vi "MQTT_PingReq.vi"(8 "error in (no error)":errorcluster, 11 "SSL_Connection":T1) -> (0 "error out":errorcluster, 2 "PingReq Message":u8[](array[numeric]) format="%x", 3 "SSL_Connection":T1)   [LabVIEW 2018, in "AWS_IoT.lvlib"]
doc: "The PingReq is a ping request to the server. \n\n© 2015 - daq.io, LLC - Peter Adelhardt"
uses:
  AWS_IoT.lvlib
  Controls/SSL_Connection.ctl
  Controls/MessageType.ctl
  Controls/Retain_Flag.ctl
  Controls/QoS.ctl
  Controls/DUP_Flag.ctl
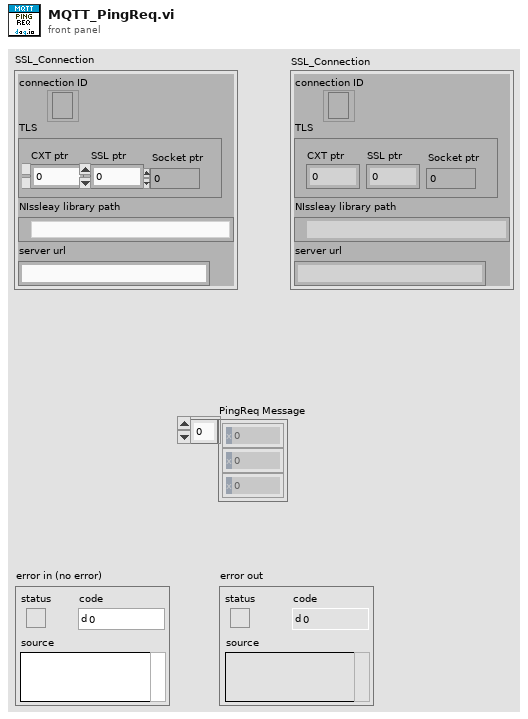
[diagram p1: front panel]
types:
  T1 = typedef "AWS_IoT.lvlib/SSL_Connection.ctl" = cluster{"connection ID":refnum<k5>, "TLS":cluster{"CXT ptr":i32, "SSL ptr":i32, "Socket ptr":i32}, "NIssleay library path":path, "server url":string}
  T2 = typedef "AWS_IoT.lvlib/DUP_Flag.ctl" = bool
  T3 = typedef "AWS_IoT.lvlib/QoS.ctl" = enum8{"At most once", "At least once", "Exactly once", "Reserved"}
  T4 = typedef "AWS_IoT.lvlib/Retain_Flag.ctl" = bool
  T5 = typedef "AWS_IoT.lvlib/MessageType.ctl" = enum32{"Reserved", "CONNECT", "CONNACK", "PUBLISH", "PUBACK", "PUBREC", "PUBREL", "PUBCOMP", "SUBSCRIBE", "SUBACK", "UNSUBSCRIBE", "UNSUBACK", "PINGREQ", "PINGRESP", "DISCONNECT", "Reserved2"}
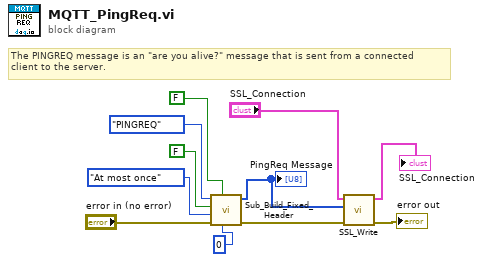
[diagram p0: block diagram]
diagram:
  # "The PINGREQ message is an \"are you alive?\" message that is sent from a connected\nclient to the server."
  n1 = call "Sub_Build_Fixed_Header.vi"("Remaining Length"=u32 0, "Retain"=T4 FALSE, "error in (no error)"="error in (no error)", "QoS"=QoS."At most once", "DUP"=T2 FALSE, "MessageType"=MessageType."PINGREQ") -> ("error out"=w5:errorcluster, "Fixed Header"=w2:u8[])  [unwired: 4 in]
  "PingReq Message" <- w2
  n2 = call "SSL_Write.vi"("error in (no error)"=w5, "data in"=w2, "SSL_Connection"="SSL_Connection") -> ("error out"=→"error out":errorcluster, "SSL_Connection"=→"SSL_Connection":T1)  [unwired: 7 in]
